vi "V-Meter Test Communications (2000).vi"(8 "error in (no error)":errorcluster, 11 "VISA resource name in":refnum<visa-resource-name>) -> (0 "error out":errorcluster, 3 "VISA resource name out":refnum<visa-resource-name>)   [LabVIEW 2016, in "Hall Effect Library.lvlib"]
uses:
  Hall Effect Library.lvlib
  <instrlib>/Keithley 2000/Keithley 2000.lvlib
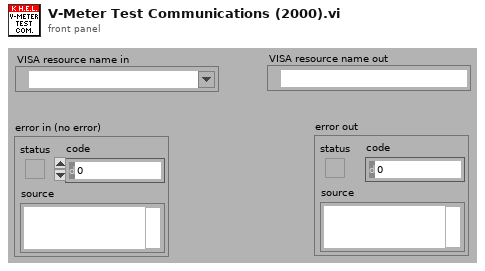
[diagram p1: front panel]
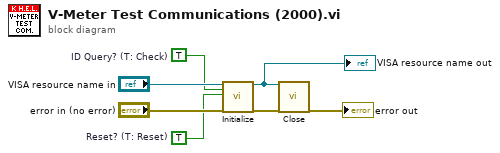
[diagram p0: block diagram]
diagram:
  w1 = TRUE  # Reset? (T: Reset)
  w2 = TRUE  # ID Query? (T: Check)
  n1 = call <instrlib>:"Initialize.vi"("VISA resource name"="VISA resource name in", "ID Query? (T: Check)"=w2, "Reset? (T: Reset)"=w1, "error in (no error)"="error in (no error)") -> ("VISA resource name out"=w3:refnum<visa-resource-name>, "error out"=w7:errorcluster)  [unwired: 14 out]
  "VISA resource name out" <- w3
  n2 = call <instrlib>:"Close.vi"("VISA resource name"=w3, "error in (no error)"=w7) -> ("error out"=→"error out":errorcluster)  [unwired: 17 out]
